vi "CRYPixel to x-y.vi"(6 "Y Scale.Range":T1, 7 "MapMode":u16(slide)=1 caption="Axis:", 8 "X Scale.Range":T1, 9 "Plot Area:Size":T2, 10 "Plot Area Bounds":T3, 11 "Graph Cordinate":cluster{"XPos":i32, "YPos":i32}) -> (2 "x-y cordinate":cluster{dbl, dbl}, 3 "abs(x)":cluster{dbl, dbl})   [LabVIEW 2013]
uses:
  <vilib>/Utility/miscctls.llb/LVRectTypeDef.ctl
  <vilib>/Utility/miscctls.llb/LVBoundsTypeDef.ctl
  <vilib>/Utility/miscctls.llb/LVRangeTypeDef.ctl
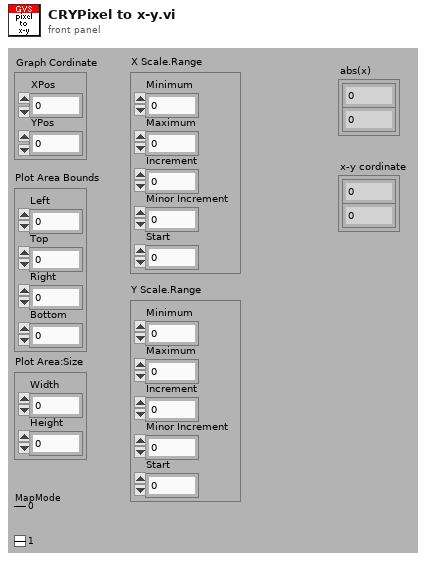
[diagram p1: front panel]
types:
  T1 = typedef "LVRangeTypeDef.ctl" = cluster{"Minimum":dbl, "Maximum":dbl, "Increment":dbl, "Minor Increment":dbl, "Start":dbl}
  T2 = typedef "LVBoundsTypeDef.ctl" = cluster{"Width":u32, "Height":u32}
  T3 = typedef "LVRectTypeDef.ctl" = cluster{"Left":i16, "Top":i16, "Right":i16, "Bottom":i16}
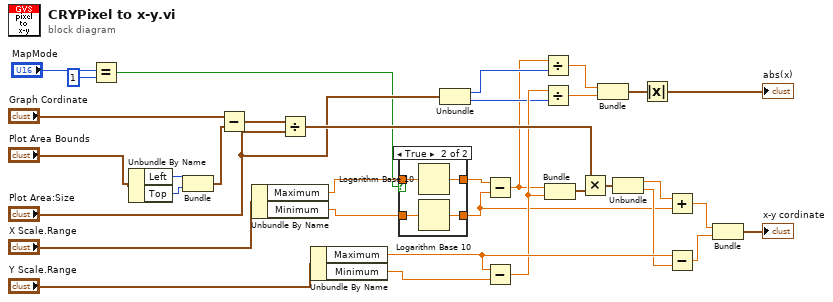
[diagram p0: block diagram]
diagram:
  n1 = Equal?(x="MapMode", y=u16 1) -> (x = y?=w1:bool)
  n2 = Unbundle By Name("Plot Area Bounds") -> ("Left"=w11:i16, "Top"=w10:i16)
  n3 = Bundle("Left"=w11, "Top"=w10) -> (w9:cluster{"Left":i16, "Top":i16})  [unwired: 1 out]
  n4 = Subtract(x="Graph Cordinate", y=w9) -> (x-y=w8:cluster{i32, i32})
  n5 = Unbundle By Name("X Scale.Range") -> ("Maximum"=w16:dbl, "Minimum"=w15:dbl)
  n6 = Divide(x=w8, y="Plot Area:Size") -> (x/y=w34:cluster{dbl, dbl})
  n7 = Unbundle By Name("Y Scale.Range") -> ("Maximum"=w29:dbl, "Minimum"=w32:dbl)
  n8 = case shown="True" w1 {
    tunnel: [w35 w40] -> w19
    tunnel: [w36 w39] -> w18
    tunnel: w16 -> [w36 w38]
    tunnel: w15 -> [w35 w37]
    frame False {
    }
    frame True {
      n9 = Logarithm Base 10(1:w38) -> (0:w39:dbl)
      n10 = Logarithm Base 10(1:w37) -> (0:w40:dbl)
    }
  }
  n11 = Unbundle("Plot Area:Size") -> ("Width"=w24:u32, "Height"=w25:u32)
  n12 = Subtract(x=w18, y=w19) -> (x-y=w14:dbl)
  n13 = Subtract(x=w29, y=w32) -> (x-y=w26:dbl)
  n14 = Divide(x=w14, y=w24) -> (x/y=w22:dbl)
  n15 = Divide(x=w26, y=w25) -> (x/y=w23:dbl)
  n16 = Bundle(w14, w26) -> (w33:cluster{dbl, dbl})  [unwired: 1 out]
  n17 = Multiply(x=w34, y=w33) -> (x*y=w31:cluster{dbl, dbl})
  n18 = Bundle(w22, w23) -> (w21:cluster{dbl, dbl})  [unwired: 1 out]
  n19 = Unbundle(w31) -> (w30:dbl, w28:dbl)
  n20 = Absolute Value(x=w21) -> (abs(x)=→"abs(x)":cluster{dbl, dbl})
  n21 = Add(x=w30, y=w19) -> (x+y=w13:dbl)
  n22 = Subtract(x=w29, y=w28) -> (x-y=w27:dbl)
  n23 = Bundle(w13, w27) -> (→"x-y cordinate":cluster{dbl, dbl})  [unwired: 1 out]
